vi "GetRoom.vi"(7 "LabVIEW Web Service Request":refnum<class "Web Request.lvclass">, 9 "Command":string, 10 "Room":i32) -> (2 "Response":string)   [LabVIEW 2015]
uses:
  <vilib>/wsapi/Web Request.lvclass
  TypeDef/RoomsActionEnum.ctl
panel:
  out "current time":timestamp
  out "postdata":string
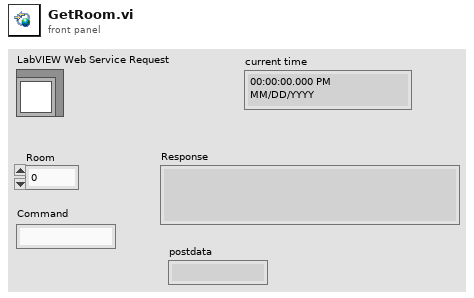
[diagram p1: front panel]
types:
  T1 = typedef "RoomsActionEnum.ctl" = enum16{"Init", "Add Room", "Remove Room", "Read Room", "Read Flag", "Read Flag State", "Write Flag State", "Read Flag Color", "Write Flag Color", "Read Bed Vacant", "Write Bed Vacant", "Read Personnel", "Add Personnel", "Remove Personnel", "Read Requests", "Add Request", "Remove Request", "Read Beacon ID", "Write Beacon ID", "Write Bed URL", "Read Bed URL", "Read Rooms Numbers", "Write Flag"}
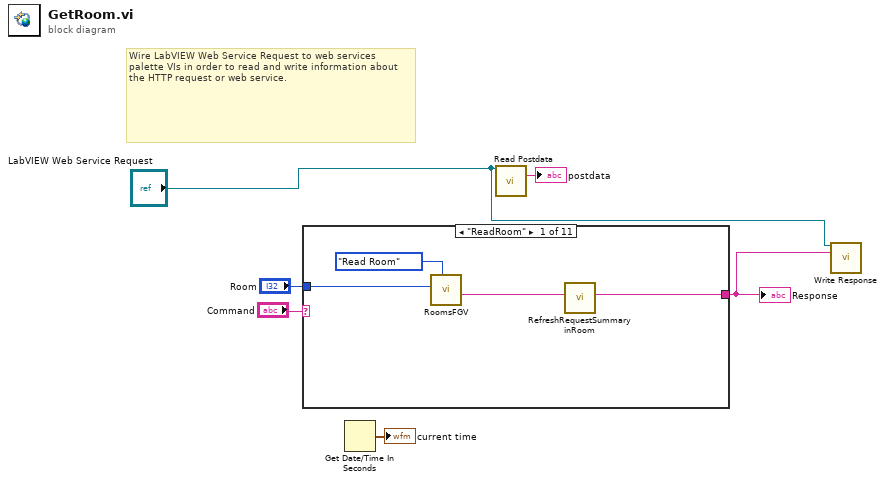
[diagram p0: block diagram]
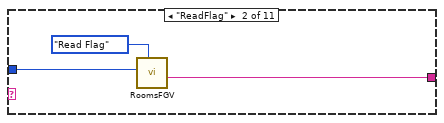
[diagram p2: hidden frame]
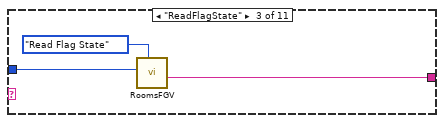
[diagram p3: hidden frame]
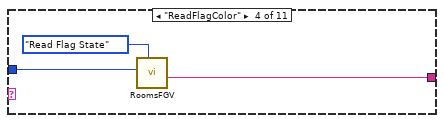
[diagram p4: hidden frame]
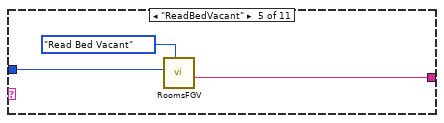
[diagram p5: hidden frame]
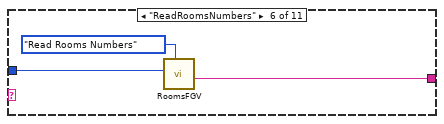
[diagram p6: hidden frame]
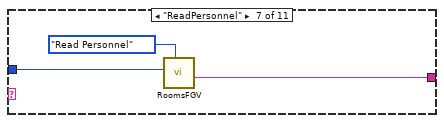
[diagram p7: hidden frame]
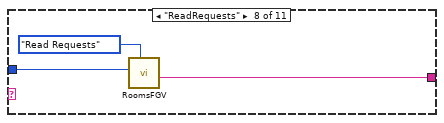
[diagram p8: hidden frame]
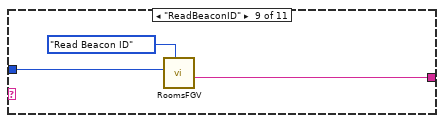
[diagram p9: hidden frame]
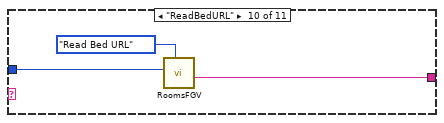
[diagram p10: hidden frame]
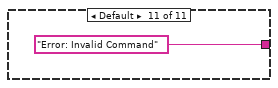
[diagram p11: hidden frame]
diagram:
  # "Wire LabVIEW Web Service Request to web services palette VIs in order to read and write information about the HTTP request or web service."
  n1 = case shown="\"ReadRoom\"" "Command" {
    tunnel: "Room" -> [w9 w12 w15 w18 w21 w25 w27 w30 w33 w36 _]
    tunnel: [w7 w11 w14 w17 w20 w24 w26 w29 w32 w35 "Error: Invalid Command" ("Data Out")] -> w3
    frame "ReadRoom" {
      n2 = call "RoomsFGV.vi"("Actions"=RoomsActionEnum."Read Room", "Room"=w9) -> ("Data Out"=w8:string)  [unwired: 8 in, 1 out]
      n3 = call "RefreshRequestSummaryinRoom.vi"("Room"=w8) -> ("Fresh Room"=w7:string)  [unwired: 9 in, 1 out]
    }
    frame "ReadFlag" {
      n4 = call "RoomsFGV.vi"("Actions"=RoomsActionEnum."Read Flag", "Room"=w12) -> ("Data Out"=w11:string)  [unwired: 8 in, 1 out]
    }
    frame "ReadFlagState" {
      n5 = call "RoomsFGV.vi"("Actions"=RoomsActionEnum."Read Flag State", "Room"=w15) -> ("Data Out"=w14:string)  [unwired: 8 in, 1 out]
    }
    frame "ReadFlagColor" {
      n6 = call "RoomsFGV.vi"("Actions"=RoomsActionEnum."Read Flag State", "Room"=w18) -> ("Data Out"=w17:string)  [unwired: 8 in, 1 out]
    }
    frame "ReadBedVacant" {
      n7 = call "RoomsFGV.vi"("Actions"=RoomsActionEnum."Read Bed Vacant", "Room"=w21) -> ("Data Out"=w20:string)  [unwired: 8 in, 1 out]
    }
    frame "ReadRoomsNumbers" {
      n8 = call "RoomsFGV.vi"("Actions"=RoomsActionEnum."Read Rooms Numbers", "Room"=w25) -> ("Data Out"=w24:string)  [unwired: 8 in, 1 out]
    }
    frame "ReadPersonnel" {
      n9 = call "RoomsFGV.vi"("Actions"=RoomsActionEnum."Read Personnel", "Room"=w27) -> ("Data Out"=w26:string)  [unwired: 8 in, 1 out]
    }
    frame "ReadRequests" {
      n10 = call "RoomsFGV.vi"("Actions"=RoomsActionEnum."Read Requests", "Room"=w30) -> ("Data Out"=w29:string)  [unwired: 8 in, 1 out]
    }
    frame "ReadBeaconID" {
      n11 = call "RoomsFGV.vi"("Actions"=RoomsActionEnum."Read Beacon ID", "Room"=w33) -> ("Data Out"=w32:string)  [unwired: 8 in, 1 out]
    }
    frame "ReadBedURL" {
      n12 = call "RoomsFGV.vi"("Actions"=RoomsActionEnum."Read Bed URL", "Room"=w36) -> ("Data Out"=w35:string)  [unwired: 8 in, 1 out]
    }
    frame Default {
    }
  }
  "Response" <- w3
  n13 = Get Date/Time In Seconds() -> (seconds since 1Jan1904=→"current time":timestamp)
  n14 = call <vilib>:"Read Postdata.vi"("LabVIEW Web Service Request"="LabVIEW Web Service Request") -> ("postdata"=→"postdata":string)  [unwired: 12 in, 2 out]
  n15 = call <vilib>:"Write Response.vi"("LabVIEW Web Service Request"="LabVIEW Web Service Request", "response string"=w3) -> ()  [unwired: 12 in, 2 out]
